vi "AddGlyphtoGManager.vi"(8 "error in":errorcluster, 10 "glyph manager":T1, 11 "NISE_CEF_Node in":refnum<class "NISE_CEF_Node.lvclass">) -> (0 "error out":errorcluster, 2 "glyph manager out":T1, 3 "NISE_CEF_Node out":refnum<class "NISE_CEF_Node.lvclass">)   [LabVIEW 2013, in "NISE_CEF_Node.lvclass"]
uses:
  NISE_CEF_Node.lvclass
  glyph manager/glyph manager.ctl
  <vilib>/picture/picture.llb/imagedata.ctl
  glyph manager/glyph manager.lvlib
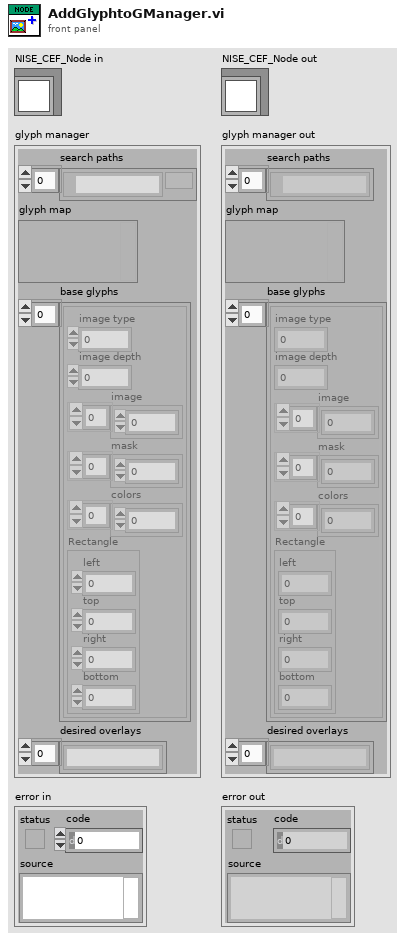
[diagram p1: front panel]
types:
  T1 = typedef "glyph manager.lvlib/glyph manager.ctl" = cluster{"search paths":path[], "glyph map":variant, "base glyphs":T2[], "desired overlays":string[]}
  T2 = typedef "imagedata.ctl" = cluster{"image type":i32, "image depth":i32, "image":u8[], "mask":u8[], "colors":u32[], "Rectangle":cluster{"left":i16, "top":i16, "right":i16, "bottom":i16}}
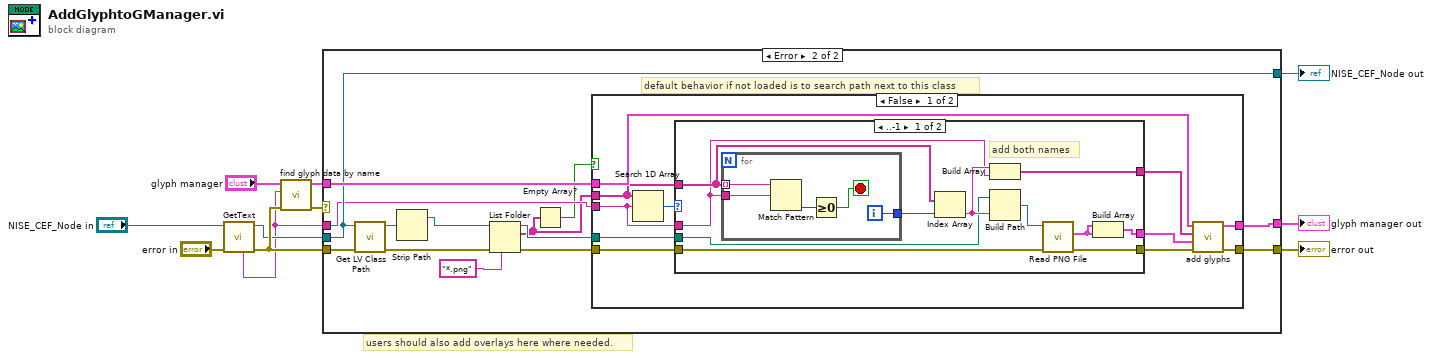
[diagram p0: block diagram]
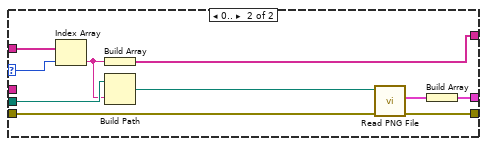
[diagram p3: hidden frame]
diagram:
  # "users should also add overlays here where needed."
  n1 = call-dynamic "GetText.vi"("error in"="error in", "node in"="NISE_CEF_Node in") -> ("error out"=w4:errorcluster, "node out"=w3:refnum<class "NISE_CEF_Node.lvclass">, "glyph"=w1:string)  [unwired: 5 in, 2 out]
  n2 = call "find glyph data by name.vi"("error in"=w4, "name"=w1, "glyph manager in"="glyph manager") -> ("error out"=w9:errorcluster, "glyph manager out"=w7:T1)  [unwired: 5 in, 2 out]
  n3 = case shown="Error" w9 {
    selector: w9 -> [w14 _]
    tunnel: [w14 w21] -> w8
    tunnel: w4 -> [_ w28]
    tunnel: w7 -> [w13 w19]
    tunnel: [w13 w20] -> w6
    tunnel: w3 -> [w12 w18]
    tunnel: [w12 w18] -> w2
    tunnel: w1 -> [_ w17]
    frame No Error {
      # "already loaded/backwards compat"
    }
    frame Error {
      # "default behavior if not loaded is to search path next to this class"
      n4 = call <vilib>:"Get LV Class Path.vi"("error in (no error)"=w28, "object"=w18) -> ("error out"=w26:errorcluster, "class path"=w27:path)  [unwired: 8 in]
      n5 = Strip Path(path=w27) -> (stripped path=w25:path)  [unwired: 1 out]
      n6 = List Folder(path=w25, pattern="*.png", error in=w26) -> (path out=w23:path, filenames=w16:string[], error out=w22:errorcluster)  [unwired: 1 in, 1 out]
      n7 = Empty Array?(array=w16) -> (empty?=w15:bool)
      n8 = case shown="False" w15 {
        tunnel: w23 -> [w38 _]
        tunnel: w22 -> [w37 w66]
        tunnel: [w35 w66] -> w21
        tunnel: [w34 w67] -> w20
        tunnel: w19 -> [w33 w67]
        tunnel: w17 -> [w30 _]
        tunnel: w16 -> [w29 _]
        frame False {
          n9 = Search 1D Array(1D array=w29, element=w30) -> (index of element=w39:i32)  [unwired: 1 in]
          n10 = case shown="..-1" w39 {
            selector: w39 -> [_ w64]
            tunnel: w38 -> [w48 w63]
            tunnel: w29 -> [w47 w65]
            tunnel: w37 -> [w45 w61]
            tunnel: [w40 w58] -> w36
            tunnel: [w41 w57] -> w32
            tunnel: [w43 w56] -> w31
            tunnel: w30 -> [w44 _]
            frame ..-1 {
              # "add both names"
              n11 = for {
                tunnel: w47 -> [w55] mode=indexing
                tunnel: w44 -> [w54]
                tunnel: [w51] -> w46
                i -> [w51]
                stop <- w52 stop-if-true
                n12 = Match Pattern(string=w55, regular expression=w54) -> (offset past match=w53:i32)  [unwired: 1 in, 3 out]
                n13 = Greater Or Equal To 0?(x=w53) -> (x >= 0?=w52:bool)
              }
              n14 = Index Array(array=w47, index=w46) -> (element=w50:string)
              n15 = Build Array(w50, w44) -> (w41:string[])
              n16 = Build Path(base path=w48, name or relative path=w50) -> (appended path=w49:path)
              n17 = call <vilib>:"Read PNG File.vi"("error in (no error)"=w45, "path to PNG file"=w49) -> ("error out"=w40:errorcluster, "image data"=w42:T2)  [unwired: 7 in, 1 out]
              n18 = Build Array(w42, w42) -> (w43:T2[])
            }
            frame 0.. {
              n19 = Index Array(array=w65, index=w64) -> (element=w62:string)
              n20 = Build Array(w62) -> (w57:string[])
              n21 = Build Path(base path=w63, name or relative path=w62) -> (appended path=w60:path)
              n22 = call <vilib>:"Read PNG File.vi"("error in (no error)"=w61, "path to PNG file"=w60) -> ("error out"=w58:errorcluster, "image data"=w59:T2)  [unwired: 7 in, 1 out]
              n23 = Build Array(w59) -> (w56:T2[])
            }
          }
          n24 = call "add glyphs.vi"("error in"=w36, "glyphs"=w31, "names"=w32, "glyph manager in"=w33) -> ("error out"=w35:errorcluster, "glyph manager out"=w34:T1)  [unwired: 6 in]
        }
        frame True {
        }
      }
    }
  }
  "error out" <- w8
  "NISE_CEF_Node out" <- w2
  "glyph manager out" <- w6
